vi "String to Array of Floats.vi"(1 "String":string) -> (0 "Array of floats":dbl[](array[numeric]))   [LabVIEW 2017, in "Drivers.lvlib" / "ASI TG-1000.lvlib"]
uses:
  ASI TG-1000.lvlib
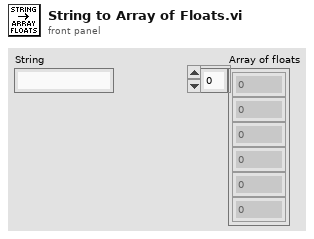
[diagram p1: front panel]
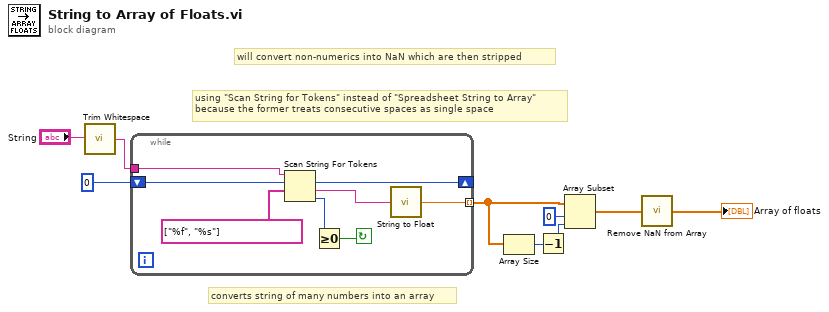
[diagram p0: block diagram]
diagram:
  # "will convert non-numerics into NaN which are then stripped"
  # "using \"Scan String for Tokens\" instead of \"Spreadsheet String to Array\"\nbecause the former treats consecutive spaces as single space"
  # "converts string of many numbers into an array"
  n1 = call <vilib>:"Trim Whitespace.vi"("string"="String") -> ("trimmed string"=w9:string)  [unwired: 1 in]
  n2 = while {
    shift-right: [w17] -> _
    shift-left: 0 ("offset past token") -> [w16]
    tunnel: w9 -> [w15]
    tunnel: [w10] -> w3 mode=indexing
    stop <- w12 continue-if-true
    n3 = Scan String For Tokens(7:string[] ["%f", "%s"] ("operators (none)"), 8:w16, 9:w15) -> (0:w14:i32, 1:w11:string, 2:w17:i32)  [unwired: 3 in, 1 out]
    n4 = Greater Or Equal To 0?(x=w14) -> (x >= 0?=w12:bool)
    n5 = call "String to Float.vi"("string"=w11) -> ("float"=w10:dbl)
  }
  n6 = Array Size(array=w3) -> (size(s)=w6:i32)
  n7 = Decrement(x=w6) -> (x-1=w5:i32)
  n8 = Array Subset(array=w3, index=0, length=w5) -> (w2:dbl[])
  n9 = call "Remove NaN from Array.vi"("Input array"=w2) -> ("Array with values deleted"=→"Array of floats":dbl[])
